vi "Wait State Timer.vi"(6 "Check Wait Rate":i32=-1, 8 "error in (no error)":errorcluster, 9 "Wait Time (Decimal String)":string, 10 "Current State":string) -> (0 "error out":errorcluster, 1 "Wait Timer Elapsed":bool, 2 "States to Enqueue":string, 4 "Time Remaining":u32)   [LabVIEW 2013]
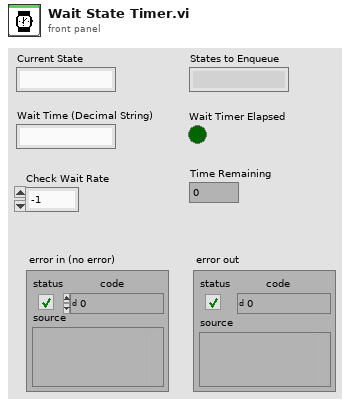
[diagram p1: front panel]
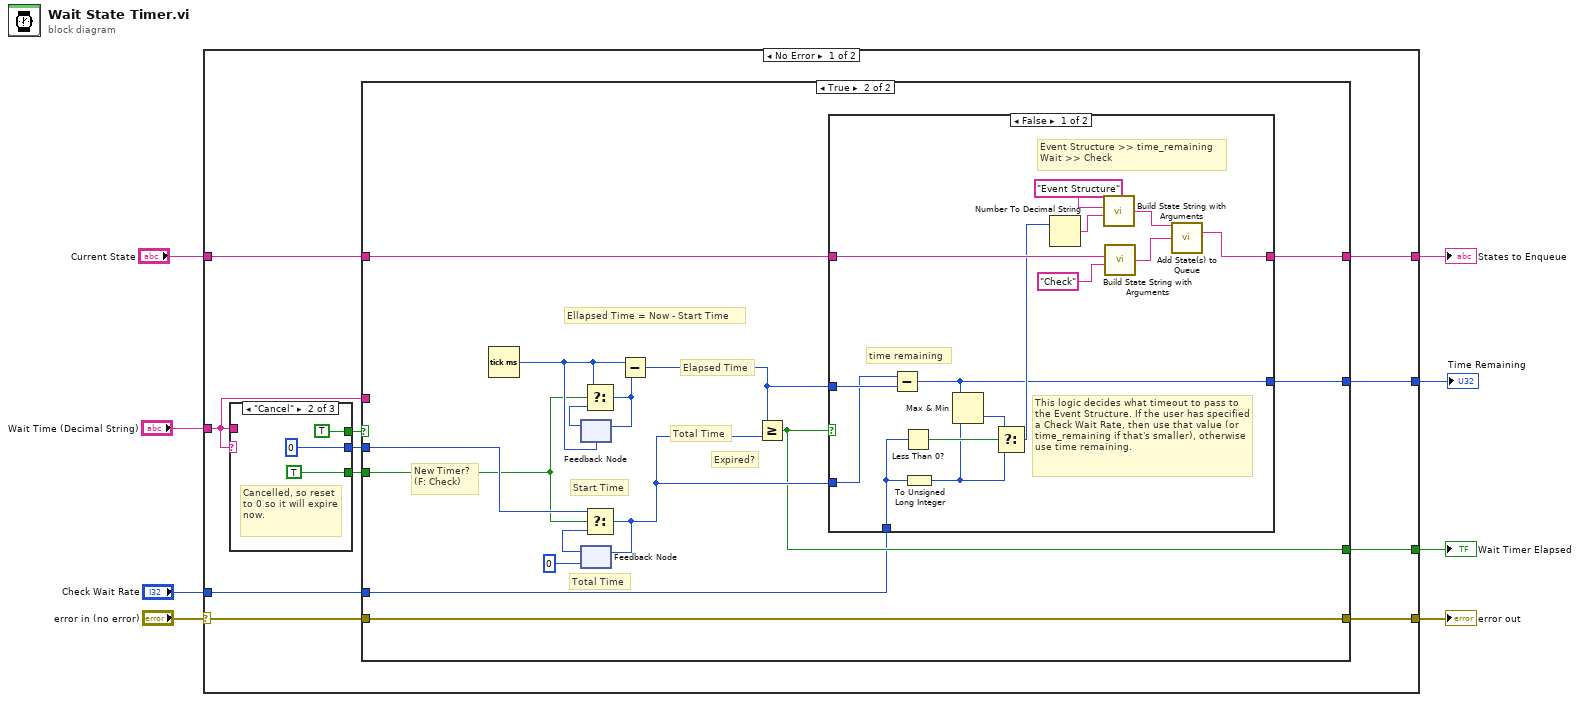
[diagram p0: block diagram]
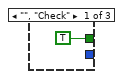
[diagram p2: hidden frame]
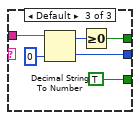
[diagram p3: hidden frame]
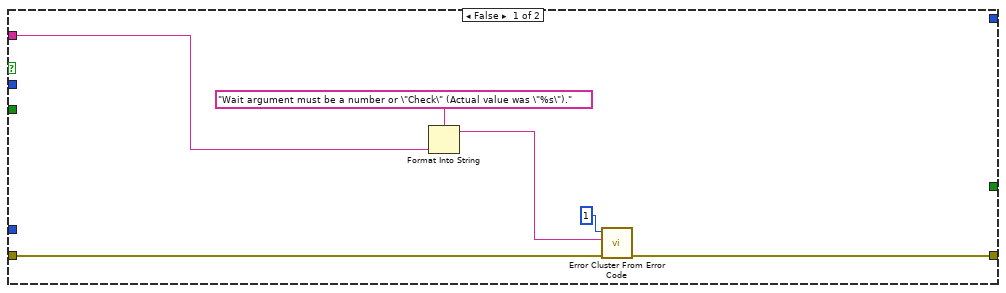
[diagram p4: hidden frame]
diagram:
  n1 = case shown="No Error" "error in (no error)" {
    selector: "error in (no error)" -> [w13 w66]
    tunnel: [w19 _] -> w8
    tunnel: "Wait Time (Decimal String)" -> [w11 _]
    tunnel: "Current State" -> [w17 _]
    tunnel: [w16 _] -> w5
    tunnel: [w14 _] -> w4
    tunnel: [w12 w66] -> w3
    tunnel: "Check Wait Rate" -> [w9 _]
    frame No Error {
      n2 = case shown="\"Cancel\"" w11 {
        tunnel: [_ u32 0 ("default (0 I32)") w29] -> w18
        tunnel: [TRUE TRUE w26] -> w15
        tunnel: w11 -> [_ _ w25]
        tunnel: [_ TRUE TRUE] -> w10
        frame "", "Check" {
        }
        frame "Cancel" {
          # "Cancelled, so reset to 0 so it will expire now."
        }
        frame Default {
          n3 = Decimal String To Number(string=w25, default (0L)=u32 0 ("default (0 I32)")) -> (offset past number=w27:i32, number=w29:u32)  [unwired: 1 in]
          n4 = Greater Or Equal To 0?(x=w27) -> (x >= 0?=w26:bool)
        }
      }
      n5 = case shown="True" w15 {
        tunnel: [_ w39] -> w19
        tunnel: w18 -> [_ w48]
        tunnel: w17 -> [_ w40]
        tunnel: [_ w38] -> w16
        tunnel: [_ w42] -> w14
        tunnel: [w34 w41] -> w12
        tunnel: w13 -> [w35 w41]
        tunnel: w11 -> [w32 _]
        tunnel: w10 -> [_ w37]
        tunnel: w9 -> [_ w36]
        frame False {
          n6 = Format Into String(format string="Wait argument must be a number or \"Check\" (Actual value was \"%s\").", w32) -> (resulting string=w30:string)  [unwired: 2 in, 1 out]
          n7 = call <vilib>:"Error Cluster From Error Code.vi"("error in (no error)"=w35, "error message (\"\")"=w30, "error code (0)"=1) -> ("error out"=w34:errorcluster)  [unwired: 6 in]
        }
        frame True {
          # "Total Time"
          # "Ellapsed Time = Now - Start Time"
          # "Expired?"
          # "Elapsed Time"
          # "Start Time"
          # "Total Time"
          # "New Timer?\n(F: Check)"
          n8 = Tick Count (ms)() -> (millisecond timer value=w44:u32)
          n9 = feedback #1(w44) -> (w50:u32)
          n10 = feedback #2(u32 0) -> (w49:u32)
          n11 = Select(t=w44, s=w37, f=w50) -> (s? t:f=w47:u32)
          n12 = feedback-in #1(w47) -> ()
          n13 = Select(t=w48, s=w37, f=w49) -> (s? t:f=w46:u32)
          n14 = feedback-in #2(w46) -> ()
          n15 = Subtract(x=w44, y=w47) -> (x-y=w43:u32)
          n16 = Greater Or Equal?(x=w43, y=w46) -> (x >= y?=w38:bool)
          n17 = case shown="False" w38 {
            tunnel: w46 -> [w54 _]
            tunnel: [w53 _] -> w42
            tunnel: w43 -> [w65 _]
            tunnel: w40 -> [w59 _]
            tunnel: [w58 _] -> w39
            tunnel: w36 -> [w55 _]
            frame False {
              # "This logic decides what timeout to pass to the Event Structure. If the user has specified a Check Wait Rate, then use that value (or time_remaining if that's smaller), otherwise use time remaining."
              # "time remaining"
              # "Event Structure >> time_remaining\nWait >> Check"
              n18 = Subtract(x=w54, y=w65) -> (x-y=w53:u32)
              n19 = Less Than 0?(x=w55) -> (x < 0?=w57:bool)
              n20 = To Unsigned Long Integer(number=w55) -> (unsigned 32bit integer=w52:u32)
              n21 = Max & Min(x=w53, y=w52) -> (min(x,y)=w51:u32)  [unwired: 1 out]
              n22 = Select(t=w51, s=w57, f=w52) -> (s? t:f=w56:u32)
              n23 = Number To Decimal String(number=w56) -> (decimal integer string=w61:string)  [unwired: 1 in]
              n24 = call "Build State String with Arguments.vi"("Arguments (\"\")"=w61, "State"="Event Structure") -> ("State with Arguments"=w62:string)  [unwired: 4 in]
              n25 = call "Build State String with Arguments.vi"("Arguments (\"\")"="Check", "State"=w59) -> ("State with Arguments"=w63:string)  [unwired: 4 in]
              n26 = call "Add State(s) to Queue.vi"("State(s) in Front (\"\")"=w62, "State(s) at Back (\"\")"=w63) -> ("States Out"=w58:string)  [unwired: 13 in]
            }
            frame True {
            }
          }
        }
      }
    }
    frame Error {
    }
  }
  "Wait Timer Elapsed" <- w5
  "States to Enqueue" <- w8
  "error out" <- w3
  "Time Remaining" <- w4
